vi "Read ResponseHeader.vi"(8 "error in (no error)":errorcluster, 11 "REST Client Headers_NET in":refnum<class "REST Client Headers_NET.lvclass">) -> (0 "error out":errorcluster, 2 "LabVIEWHTTPClient_NET.lvlib:HttpHeaders_Response.lvclass":refnum<class "HttpHeaders_Response.lvclass">, 3 "REST Client Headers_NET out":refnum<class "REST Client Headers_NET.lvclass">)   [LabVIEW 2018, in "REST Client_NET.lvlib" / "REST Client Headers_NET.lvclass"]
uses:
  REST Client Headers_NET.lvclass
  HttpHeaders_response/HttpHeaders_Response.lvclass
  REST Client Headers_NET.lvclass/REST Client Headers_NET.ctl
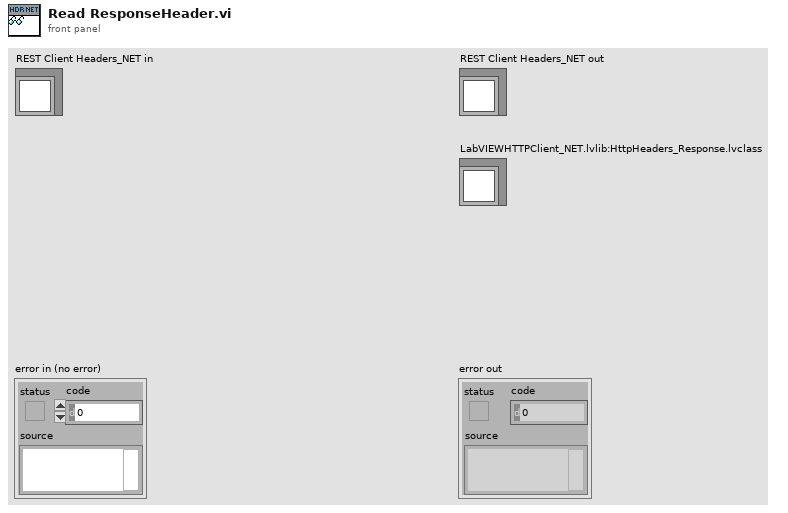
[diagram p1: front panel]
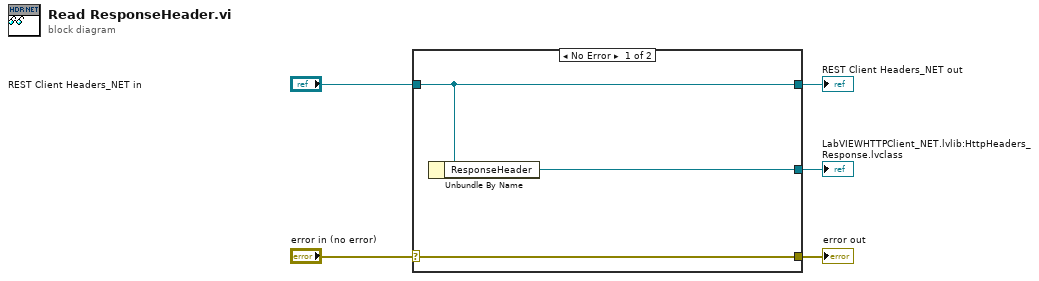
[diagram p0: block diagram]
diagram:
  n1 = case shown="No Error" "error in (no error)" {
    selector: "error in (no error)" -> [w8 w9]
    tunnel: [w8 w9] -> w4
    tunnel: [w7 w10] -> w2
    tunnel: "REST Client Headers_NET in" -> [w7 w10]
    tunnel: [w6 _] -> w1
    frame No Error {
      n2 = Unbundle By Name(w7) -> ("ResponseHeader"=w6:refnum<class "HttpHeaders_Response.lvclass">)
    }
    frame Error {
    }
  }
  "error out" <- w4
  "REST Client Headers_NET out" <- w2
  "LabVIEWHTTPClient_NET.lvlib:HttpHeaders_Response.lvclass" <- w1
